vi "SerializeMessage.vi"(7 "MsgSerializer":refnum<class "MsgSerializer.lvclass">, 9 "error in (no error)":errorcluster, 10 "Value":variant, 11 "TestManagerMsg.Measurement in":refnum<class "TestManagerMsg.Measurement.lvclass">) -> (1 "error out":errorcluster, 3 "Serialized Message":string)   [LabVIEW 2020, in "Caraya.lvlib" / "TestManagerMsg.Measurement.lvclass"]
uses:
  TestManagerMsg.Measurement.lvclass
  MsgSerializer/MsgSerializer.lvclass
  TestManagerMsg.Measurement.lvclass/TestManagerMsg.Measurement.ctl
  Test Manager Message/TestManagerMsg.lvclass
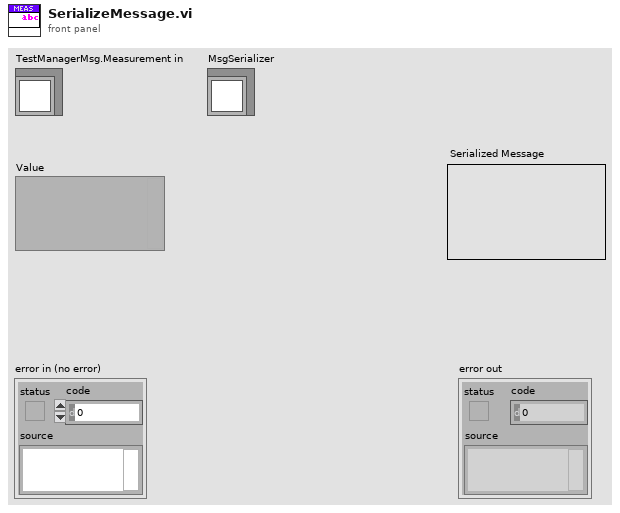
[diagram p1: front panel]
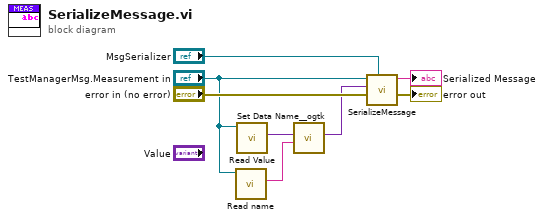
[diagram p0: block diagram]
diagram:
  n1 = call "Read name.vi"("TestManagerMsg.Measurement in"="TestManagerMsg.Measurement in") -> ("name"=w4:string)  [unwired: 9 in, 1 out]
  n2 = call "Read Value.vi"("TestManagerMsg.Measurement in"="TestManagerMsg.Measurement in") -> ("Value"=w2:variant)  [unwired: 9 in, 1 out]
  n3 = call <userlib>:"Set Data Name__ogtk.vi"("Data Name"=w4, "Data"=w2) -> ("Renamed Data"=w1:variant)  [unwired: 8 in, 1 out]
  n4 = call-parent "SerializeMessage.vi"("MsgSerializer"="MsgSerializer", "error in (no error)"="error in (no error)", "Value"=w1, "TestManagerMsg in"="TestManagerMsg.Measurement in") -> ("error out"=→"error out":errorcluster, "Serialized Message"=→"Serialized Message":string)  [unwired: 6 in]
